vi "LINC Format String.vi"(1 "string in":string) -> (0 "string out":string)   [LabVIEW 2018, in "STEPkgDriver_LINC.lvlib"]
uses:
  STEPkgDriver_LINC.lvlib
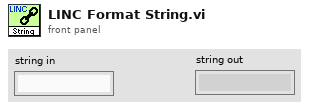
[diagram p1: front panel]
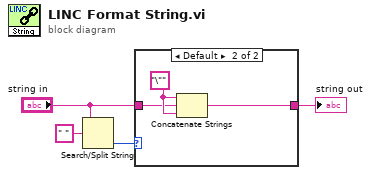
[diagram p0: block diagram]
diagram:
  n1 = Search/Split String(string="string in", search string/char (-)=" ") -> (offset of match=w3:i32)  [unwired: 1 in, 2 out]
  n2 = case shown="Default" w3 {
    tunnel: "string in" -> [w5 w7]
    tunnel: [w5 w6] -> w2
    frame -1 {
    }
    frame Default {
      w8 = "\"" ("string")
      n3 = Concatenate Strings(w8, w7, w8) -> (w6:string)
    }
  }
  "string out" <- w2
